vi "DAQmx.44xx.Get Master and Slave Tasks.vi"(8 "error in (no error)":errorcluster, 10 "AI tasks in":refnum<k21>[](array[refnum]), 11 "AI task":refnum<k21>) -> (0 "error out":errorcluster, 2 "master task":refnum<k21>, 3 "AI task out":refnum<k21>)   [LabVIEW 2019, in "DAQmx.lvclass"]
uses:
  DAQmx.lvclass
  <userlib>/_OpenG.lib/array/array.llb/Search 1D Array (U32)__ogtk.vi
  <userlib>/_OpenG.lib/array/array.llb/Index 1D Array Elements (U32)__ogtk.vi
  <resource>/objmgr/daqmx.rc
panel:
  out "x+y":i32
  out "time":dbl format="%#_6p"
  out "Slot Number":u32[](array[numeric])
  out "Chassis Number":u32[](array[numeric])
  out "Devices":tag[](array[tag])
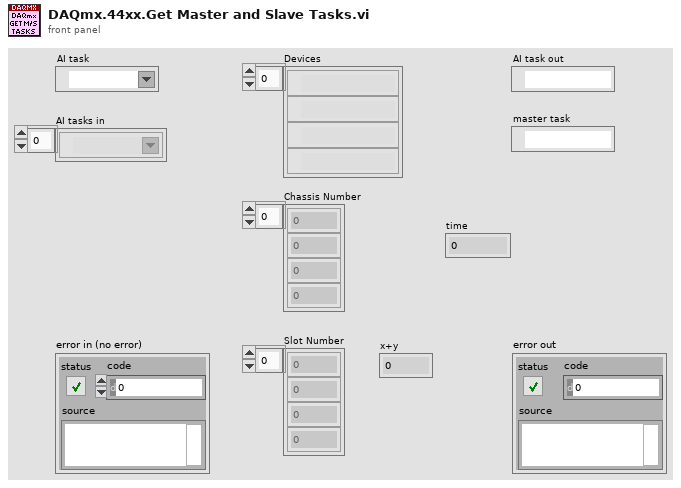
[diagram p1: front panel]
types:
  T1 = typedef "DAQmx.lvclass/DAQ.Config.Device Type--enum.ctl" = enum16{"None", "USB-4431", "PXI-446x"}
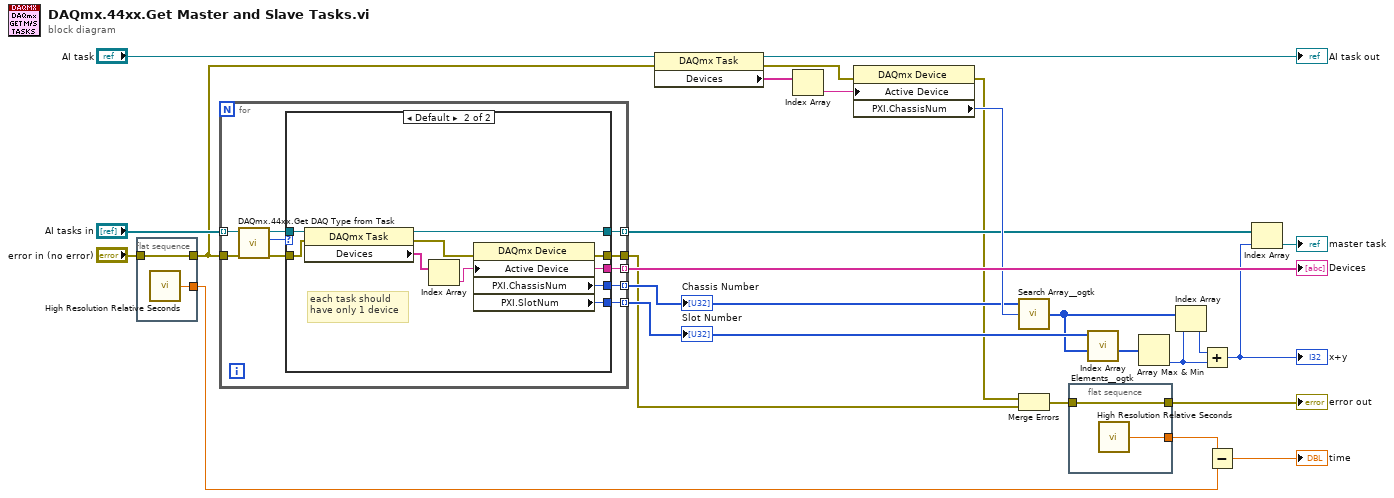
[diagram p0: block diagram]
diagram:
  n1 = flat-sequence {
    tunnel: [w28] -> w7
    tunnel: "error in (no error)" -> [w28]
    tunnel: [w27] -> w15
    frame #0 {
      n2 = call <vilib>:"High Resolution Relative Seconds.vi"() -> ("relative seconds"=w27:dbl)
    }
  }
  n3 = for {
    tunnel: "AI tasks in" -> [w32] mode=indexing
    tunnel: [w34] -> w19 mode=indexing
    tunnel: [w38] -> w9 mode=indexing
    tunnel: [w36] -> w25 mode=indexing
    tunnel: [w37] -> w22 mode=indexing
    tunnel: [w35] -> w3
    tunnel: w7 -> [w30]
    n4 = call "DAQmx.44xx.Get DAQ Type from Task.vi"("error in (no error)"=w30, "Task in"=w32) -> ("error out"=w31:errorcluster, "DAQ Type"=w29:T1, "Task out"=w33:refnum<k21>)  [unwired: 5 in, 2 out]
    n5 = case shown="Default" w29 {
      tunnel: [_ w48] -> w38
      tunnel: [_ w47] -> w37
      tunnel: [_ w46] -> w36
      tunnel: [w40 w45] -> w35
      tunnel: [w39 w44] -> w34
      tunnel: w33 -> [w39 w43]
      tunnel: w31 -> [w40 w42]
      frame "USB-4431" {
      }
      frame Default {
        # "each task should\nhave only 1 device"
        n6 = property class="DAQmx Task"(reference=w43, error in=w42) -> (reference out=w44:refnum<k21>, error out=w49:errorcluster, "Devices"=w41:tag[])
        n7 = Index Array(array=w41) -> (element=w46:tag)  [unwired: 1 in]
        n8 = property class="DAQmx Device"(error in=w49, "Active Device"=w46) -> (error out=w45:errorcluster, "PXI.ChassisNum"=w48:u32, "PXI.SlotNum"=w47:u32)  [unwired: 1 in, 1 out]
      }
    }
  }
  "Devices" <- w25
  "Chassis Number" <- w9
  "Slot Number" <- w22
  n9 = property class="DAQmx Task"(reference="AI task", error in=w7) -> (reference out=→"AI task out":refnum<k21>, error out=w24:errorcluster, "Devices"=w5:tag[])
  n10 = Index Array(array=w5) -> (element=w4:tag)  [unwired: 1 in]
  n11 = property class="DAQmx Device"(error in=w24, "Active Device"=w4) -> (error out=w6:errorcluster, "PXI.ChassisNum"=w23:u32)  [unwired: 1 in, 1 out]
  n12 = call-poly <userlib>:"Search Array__ogtk.vi"("Array"=w9, "Element Data"=w23) -> ("Indices of Elements"=w2:i32[])  [unwired: 7 in]
  n13 = Merge Errors(w6, w3) -> (w8:errorcluster)
  n14 = flat-sequence {
    tunnel: [w51] -> w17
    tunnel: w8 -> [w51]
    tunnel: [w50] -> w16
    frame #0 {
      n15 = call <vilib>:"High Resolution Relative Seconds.vi"() -> ("relative seconds"=w50:dbl)
    }
  }
  n16 = call-poly <userlib>:"Index Array Elements__ogtk.vi"("indices"=w2, "array"=w22) -> ("elements"=w21:u32[])  [unwired: 9 in]
  n17 = Array Max & Min(array=w21) -> (min index (indices)=w13:i32)  [unwired: 3 out]
  n18 = Index Array(array=w2, index=w13) -> (element=w12:i32)
  n19 = Add(x=w12, y=w13) -> (x+y=w1:i32)
  "x+y" <- w1
  n20 = Subtract(x=w16, y=w15) -> (x-y=→"time":dbl)
  n21 = Index Array(array=w19, index=w1) -> (element=→"master task":refnum<k21>)
  "error out" <- w17
